vi "listen.vi"() -> ()   [LabVIEW 2024]
uses:
  <vilib>/express/express analysis/Spectral/Block/exnSpectralBlock spectral measurements RMS poly.vi
  <vilib>/express/express analysis/Spectral/Block/exnSpectralBlock spectral measurements RMS WFM.vi
  <vilib>/express/express analysis/Spectral/XNode/ExpressSpectralMeasurementsBlockNode.xnode
  <vilib>/express/express analysis/Spectral/Block/exnSpectralBlock spectral measurements RMS DDT.vi
panel:
  out "Waveform Graph 2":dynamicdata(graph)
  in  "stop":bool
  out "Data":dynamicdata(graph)
  out "FFT - (RMS)":cluster{"f0":dbl, "df":dbl, "magnitude":dbl[]}(graph)
  out "Waveform Graph":waveform(dbl)(graph)
  in  "Array":cluster{"Freq":dbl, "phase":dbl}[](array[cluster]) {"phase" scale=0.0..180.0; "Freq" scale=0.0..1000.0}
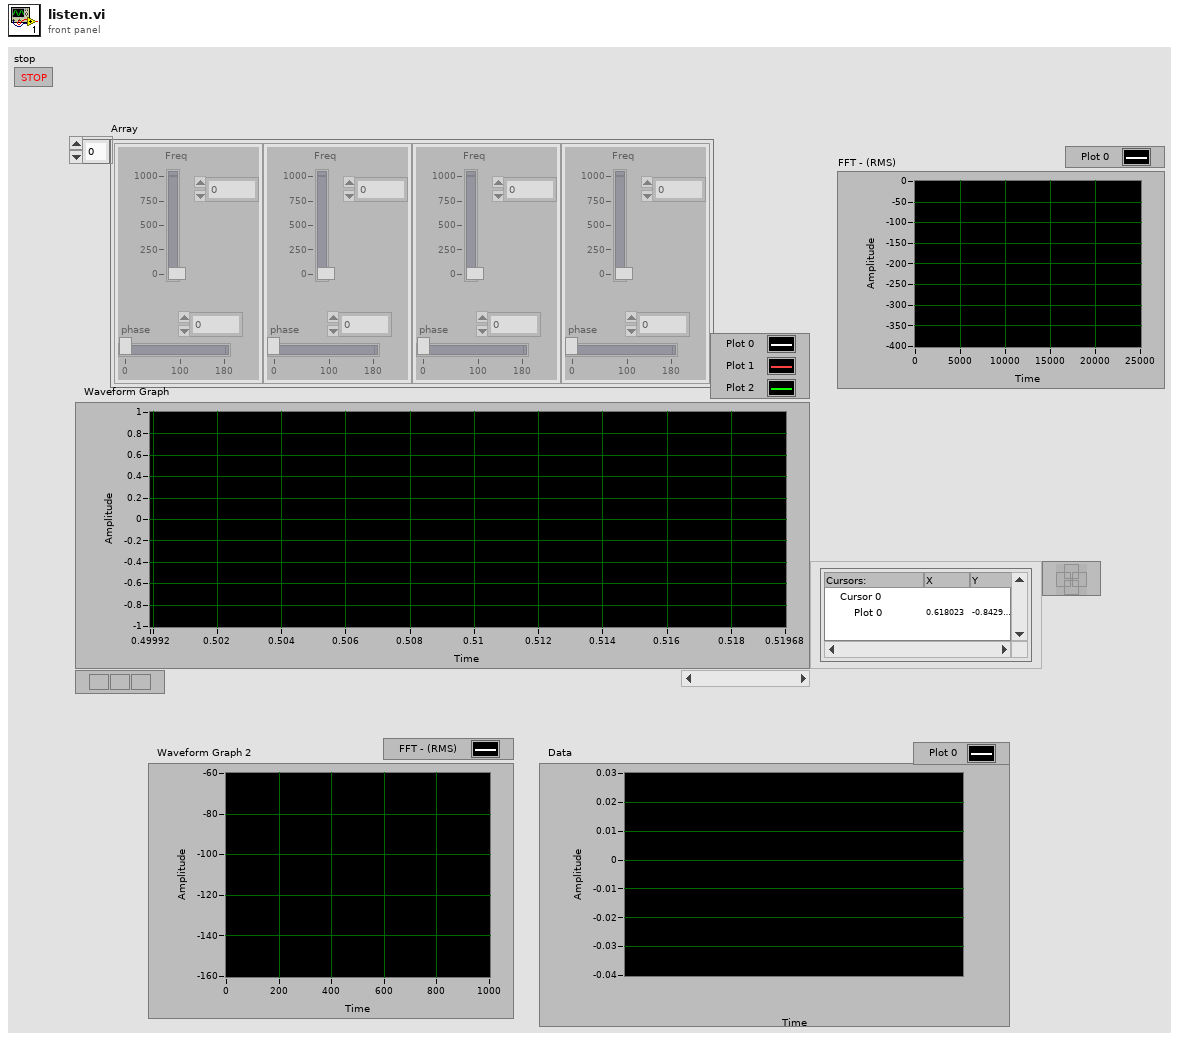
[diagram p1: front panel]
types:
  T1 = cluster{"averaging mode":u16, "weighting mode":u16, "number of averages":u32}
  T2 = cluster{"dB On (F)":bool, "unwrap phase (F)":bool, "convert to degree (F)":bool}
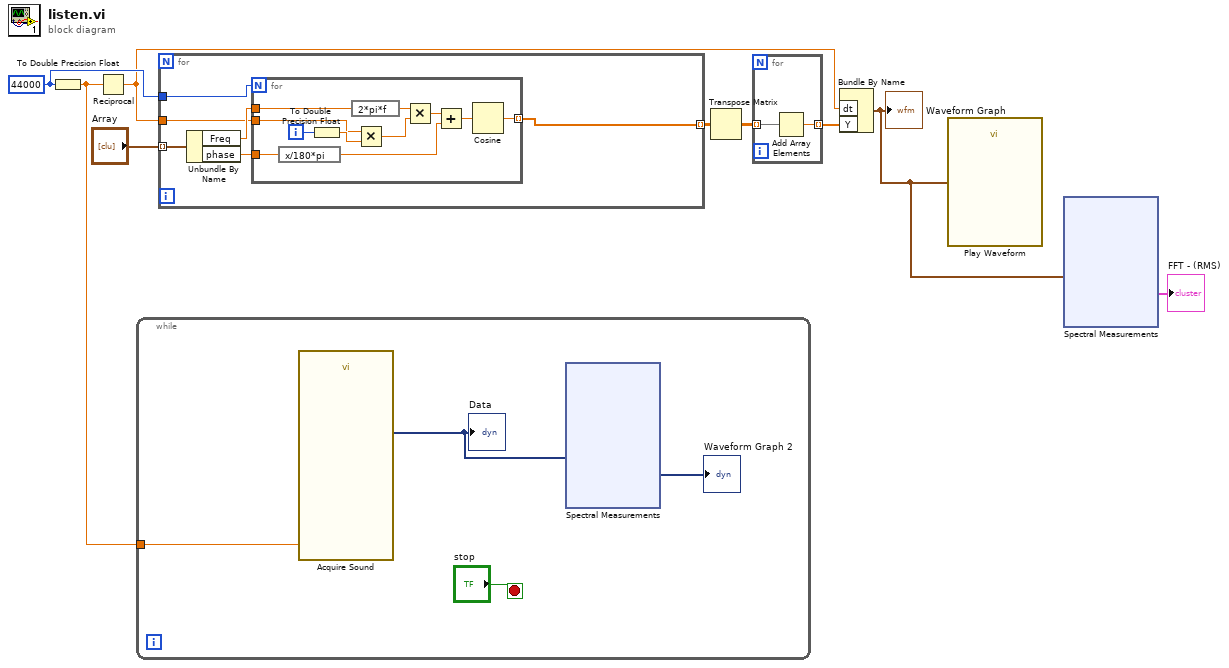
[diagram p0: block diagram]
diagram:
  w5 = 44000
  n1 = To Double Precision Float(number=w5) -> (double precision float=w1:dbl)
  n2 = Reciprocal(x=w1) -> (1/x=w4:dbl)
  n3 = while {
    tunnel: w1 -> [w12]
    stop <- "stop" stop-if-true
    n4 = call "Acquire Sound"("Sample rate (Hz)"=w12) -> ("Data"=w11:dynamicdata)  [unwired: 17 in, 1 out]
    "Data" <- w11
    n5 = xnode "Spectral Measurements"("Signals"=w11) -> ("FFT - (RMS)"=→"Waveform Graph 2":dynamicdata)  [unwired: 1 in, 2 out]
  }
  n6 = for {
    tunnel: "Array" -> [w27] mode=indexing
    tunnel: [w26] -> w8 mode=indexing
    tunnel: w5 -> [w25]
    tunnel: w4 -> [w24]
    n7 = Unbundle By Name(w27) -> ("Freq"=w29:dbl, "phase"=w28:dbl)
    n8 = for {
      N: w25 -> [_]
      tunnel: w29 -> [w40]
      tunnel: w28 -> [w39]
      tunnel: [w34] -> w26 mode=indexing
      tunnel: w24 -> [w30]
      i -> [w31]
      n9 = expression code="x/180*pi"(w39) -> (w36:dbl)
      n10 = To Double Precision Float(number=w31) -> (double precision float=w32:dbl)
      n11 = expression code="2*pi*f"(w40) -> (w38:dbl)
      n12 = Multiply(x=w30, y=w32) -> (x*y=w33:dbl)
      n13 = Multiply(x=w38, y=w33) -> (x*y=w37:dbl)
      n14 = Add(x=w37, y=w36) -> (x+y=w35:dbl)
      n15 = Cosine(x=w35) -> (cos(x)=w34:dbl)
    }
  }
  n16 = Transpose Matrix(1:w8) -> (0:w7:dbl[][])
  n17 = for {
    tunnel: [w41] -> w6 mode=indexing
    tunnel: w7 -> [w42] mode=indexing
    n18 = Add Array Elements(numeric array=w42) -> (sum=w41:dbl)
  }
  n19 = Bundle By Name("dt"=w4, "Y"=w6) -> (w3:waveform(dbl))  [unwired: 1 in]
  "Waveform Graph" <- w3
  n20 = call "Play Waveform"("Data"=w3) -> ()  [unwired: 18 in, 1 out]
  n21 = xnode "Spectral Measurements"("Signals"=w3) -> ("FFT - (RMS)"=→"FFT - (RMS)":cluster{"f0":dbl, "df":dbl, "magnitude":dbl[]})  [unwired: 1 in, 2 out]
